vi "Read Errors count.vi"(11 "Test Suite Result In":refnum<class "Test Suite Result.lvclass">) -> (1 "Error count string":string, 2 "Errors count":i32, 3 "Test Suite Result Out":refnum<class "Test Suite Result.lvclass">)   [LabVIEW 2020, in "Test Suite Result.lvclass"]
uses:
  Test Suite Result.lvclass
  Assertion Result/Public/TypeDefs/Status.ctl
  Test Suite Result.lvclass/Test Suite Result.ctl
  Test Case Result/Test Case Result.lvclass/Test Case Result.ctl
  Method Result/Method Result.lvclass/Method Result.ctl
  Test Case Result/Public/Accessors/Read Status.vi
  Test Case Result/Private/SubVIs/Merge Status.vi
  Method Result/Public/Read Status.vi
  Assertion Result/Assertion Result.lvclass
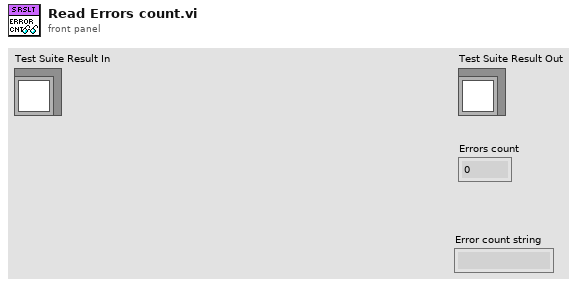
[diagram p1: front panel]
types:
  T1 = typedef "Assertion Result.lvclass/Status.ctl" = enum16{"Pass", "Fail", "Error", "Skipped", "Setup Error", "Broken", "Teardown Error"}
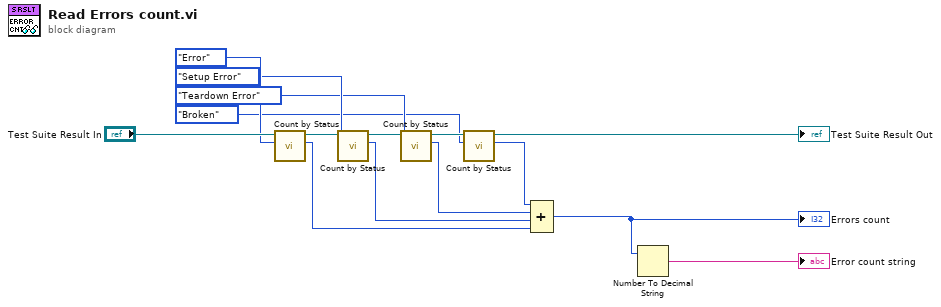
[diagram p0: block diagram]
diagram:
  n1 = call "Count by Status.vi"("Status"=Status."Error", "Test Suite Result in"="Test Suite Result In") -> ("Count"=w1:i32, "Test Suite Result out"=w14:refnum<class "Test Suite Result.lvclass">)  [unwired: 8 in]
  n2 = call "Count by Status.vi"("Status"=Status."Setup Error", "Test Suite Result in"=w14) -> ("Count"=w2:i32, "Test Suite Result out"=w13:refnum<class "Test Suite Result.lvclass">)  [unwired: 8 in]
  n3 = call "Count by Status.vi"("Status"=Status."Teardown Error", "Test Suite Result in"=w13) -> ("Count"=w3:i32, "Test Suite Result out"=w8:refnum<class "Test Suite Result.lvclass">)  [unwired: 8 in]
  n4 = call "Count by Status.vi"("Status"=Status."Broken", "Test Suite Result in"=w8) -> ("Count"=w4:i32, "Test Suite Result out"=→"Test Suite Result Out":refnum<class "Test Suite Result.lvclass">)  [unwired: 8 in]
  n5 = Compound Arithmetic op=ADD(w4, w3, w2, w1) -> (w5:i32)
  "Errors count" <- w5
  n6 = Number To Decimal String(number=w5) -> (decimal integer string=→"Error count string":string)  [unwired: 1 in]
